vi "Result To Error - Copy.vi"(8 "error in (no error)":errorcluster, 11 "Result Code":i32) -> (0 "error out":errorcluster)   [LabVIEW 2020]
doc: "Converts the result codes found in g_audio.h to a custom LabVIEW error code. The custom error code range begins at 559240."
uses:
  <vilib>/Utility/error.llb/Error Cluster From Error Code.vi
  <vilib>/ErrorRing/Error Ring.xnode
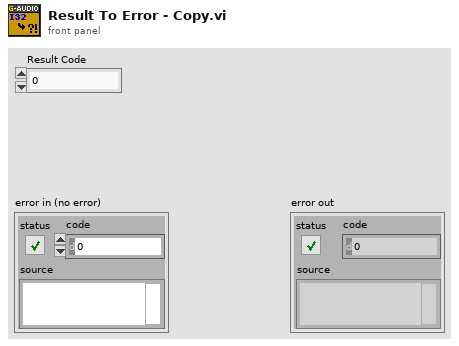
[diagram p1: front panel]
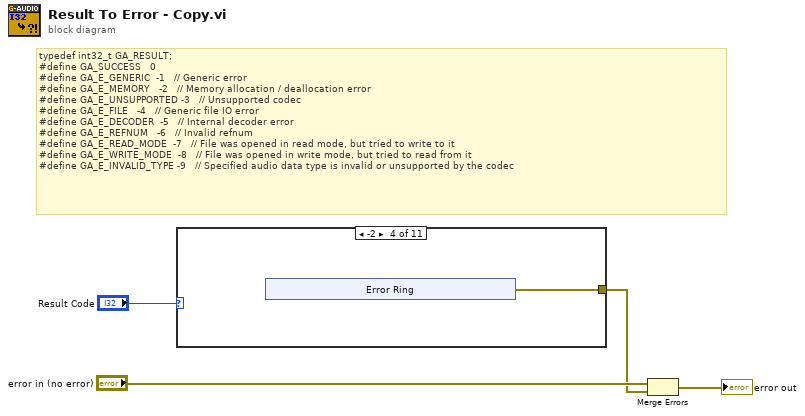
[diagram p0: block diagram]
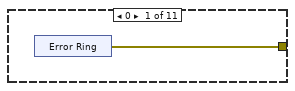
[diagram p2: hidden frame]
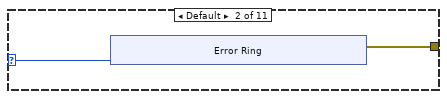
[diagram p3: hidden frame]
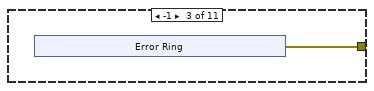
[diagram p4: hidden frame]
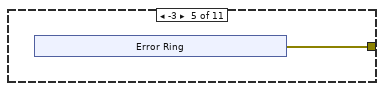
[diagram p5: hidden frame]
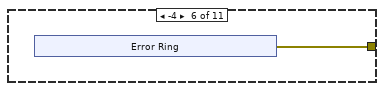
[diagram p6: hidden frame]
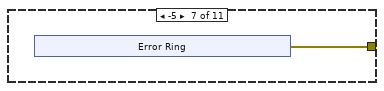
[diagram p7: hidden frame]
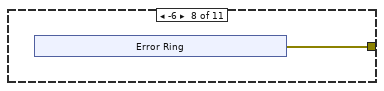
[diagram p8: hidden frame]
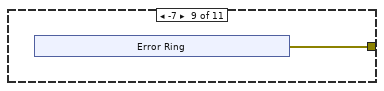
[diagram p9: hidden frame]
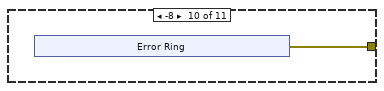
[diagram p10: hidden frame]
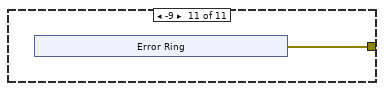
[diagram p11: hidden frame]
diagram:
  # "typedef int32_t GA_RESULT;\n#define GA_SUCCESS\t\t\t0\n#define GA_E_GENERIC\t\t-1\t\t\t// Generic error\n#define GA_E_MEMORY\t\t\t-2\t\t\t// Memory allocation / deallocation error\n#define GA_E_UNSUPPORTED\t-3\t\t\t// Unsupported codec\n#define GA_E_FILE\t\t\t-4\t\t\t// Generic file IO error\n#define GA_E_DECODER\t\t-5\t\t\t// Internal decoder error\n#define GA_E_REFNUM\t\t\t-6\t\t\t// Invalid refnum\n#define GA_E_READ_MODE\t\t-7\t\t\t// File was opened in read mode, but tried to write to it\n#define GA_E_WRITE_MODE\t\t-8\t\t\t// File was opened in write mode, but tried to read from it\n#define GA_E_INVALID_TYPE\t-9\t\t\t// Specified audio data type is invalid or unsupported by the codec"
  n1 = case shown="-2" "Result Code" {
    selector: "Result Code" -> [_ w7 _ _ _ _ _ _ _ _ _]
    tunnel: [w5 w8 w16 w22 w28 w34 w40 w46 w52 w58 w64] -> w1
    frame 0 {
      n2 = xnode "Error Ring"() -> ("error out"=w5:errorcluster)
    }
    frame Default {
      n3 = xnode "Error Ring"("parameter 0"=w7) -> ("error out"=w8:errorcluster)
    }
    frame -1 {
      n4 = xnode "Error Ring"() -> ("error out"=w16:errorcluster)
    }
    frame -2 {
      n5 = xnode "Error Ring"() -> ("error out"=w22:errorcluster)
    }
    frame -3 {
      n6 = xnode "Error Ring"() -> ("error out"=w28:errorcluster)
    }
    frame -4 {
      n7 = xnode "Error Ring"() -> ("error out"=w34:errorcluster)
    }
    frame -5 {
      n8 = xnode "Error Ring"() -> ("error out"=w40:errorcluster)
    }
    frame -6 {
      n9 = xnode "Error Ring"() -> ("error out"=w46:errorcluster)
    }
    frame -7 {
      n10 = xnode "Error Ring"() -> ("error out"=w52:errorcluster)
    }
    frame -8 {
      n11 = xnode "Error Ring"() -> ("error out"=w58:errorcluster)
    }
    frame -9 {
      n12 = xnode "Error Ring"() -> ("error out"=w64:errorcluster)
    }
  }
  n13 = Merge Errors("error in (no error)", w1) -> (→"error out":errorcluster)
